vi "Get Test Redis Client.vi"(6 "(T) Set / (F) Get":bool, 10 "Test Client In":refnum<class "Test Redis Client.lvclass">) -> (2 "Test Client Out":refnum<class "Test Redis Client.lvclass">)   [LabVIEW 2019, in "Test Redis Client for LabVIEW.lvlib"]
uses:
  Test Redis Client for LabVIEW.lvlib
  Test Redis Client/Test Redis Client.lvclass
panel:
  in  "reset (T)":bool=TRUE
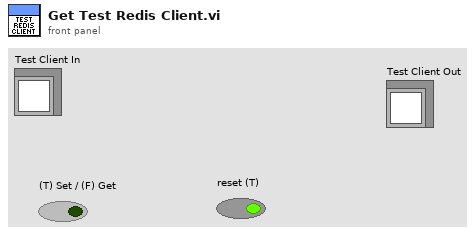
[diagram p1: front panel]
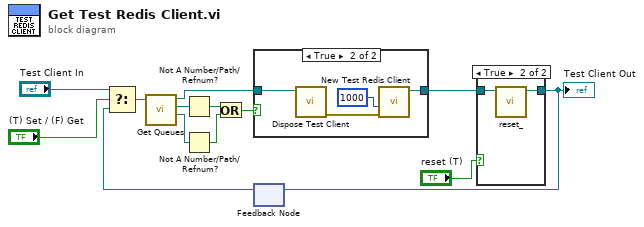
[diagram p0: block diagram]
diagram:
  n1 = feedback #1() -> (w11:refnum<class "Test Redis Client.lvclass">)  [unwired: 1 in]
  n2 = Select(t="Test Client In", s="(T) Set / (F) Get", f=w11) -> (s? t:f=w4:refnum<class "Test Redis Client.lvclass">)
  n3 = call "Get Queues.vi"("Test Redis Client in"=w4) -> ("receive queue"=w9:refnum<queue>, "send queue"=w10:refnum<queue>, "Test Redis Client out"=w5:refnum<class "Test Redis Client.lvclass">)  [unwired: 7 in, 1 out]
  n4 = Not A Number/Path/Refnum?(number/path/refnum=w10) -> (NaN/Path/Refnum?=w8:bool)
  n5 = Not A Number/Path/Refnum?(number/path/refnum=w9) -> (NaN/Path/Refnum?=w7:bool)
  n6 = Or(x=w8, y=w7) -> (x .or. y?=w6:bool)
  n7 = case shown="True" w6 {
    tunnel: w5 -> [w14 w18]
    tunnel: [w14 w15] -> w2
    frame False {
    }
    frame True {
      n8 = call "Dispose Test Client.vi"("Test Redis Client in"=w18) -> ("error out"=w17:errorcluster)  [unwired: 10 in]
      n9 = call "New Test Redis Client.vi"("error in (no error)"=w17, "timeout (ms)"=1000) -> ("Test Redis Client out"=w15:refnum<class "Test Redis Client.lvclass">)  [unwired: 6 in, 3 out]
    }
  }
  n10 = case shown="True" "reset (T)" {
    tunnel: w2 -> [w19 w21]
    tunnel: [w19 w20] -> w1
    frame False {
    }
    frame True {
      n11 = call "reset_.vi"("Test Redis Client in"=w21) -> ("Test Redis Client out"=w20:refnum<class "Test Redis Client.lvclass">)  [unwired: 7 in, 3 out]
    }
  }
  "Test Client Out" <- w1
  n12 = feedback-in #1(w1) -> ()
